vi "JAS-Color Sensor V3 Update Color Match.vi"(9 "ColorIndex":i32, 10 "Color":cluster{"R":dbl, "G":dbl, "B":dbl}, 11 "Name":string) -> ()   [LabVIEW 2019]
uses:
  JAS-ColorMatch-FGV-Cmd.ctl
  <vilib>/Rock Robotics/WPI/ThirdParty/REV Robotics/Color SensorV3/Typedef/Color Sensor V3 Color Match.ctl
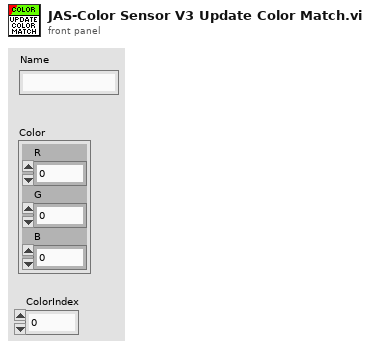
[diagram p1: front panel]
types:
  T1 = typedef "JAS-ColorMatch-FGV-Cmd.ctl" = enum16{"AddNew", "Update", "Read"}
  T2 = typedef "Color Sensor V3 Color Match.ctl" = cluster{"Name":string, "Normalized Color":cluster{"R":dbl, "G":dbl, "B":dbl}}
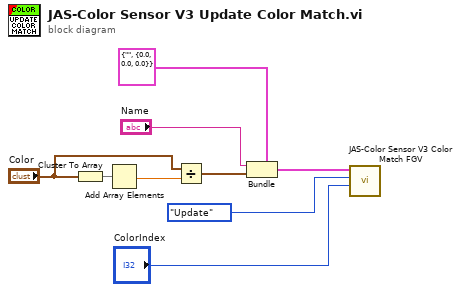
[diagram p0: block diagram]
diagram:
  n1 = Cluster To Array(cluster="Color") -> (array=w6:dbl[])
  n2 = Add Array Elements(numeric array=w6) -> (sum=w5:dbl)
  n3 = Divide(x="Color", y=w5) -> (x/y=w3:cluster{"R":dbl, "G":dbl, "B":dbl})
  n4 = Bundle(cluster=T2 {"Name"="", "Normalized Color"={"R"=0.0, "G"=0.0, "B"=0.0}} ("output cluster"), "Name"="Name", "Normalized Color"=w3) -> (w7:T2)
  n5 = call "JAS-Color Sensor V3 Color Match FGV.vi"("UpdateIndex"="ColorIndex", "ColorMatchFGV-Cmd"=JAS-ColorMatch-FGV-Cmd."Update", "Color Match"=w7) -> ()  [unwired: 7 in, 2 out]
